vi "Access2DArray.vi"(4 "Sequence Context":T1) -> (0 "error out":errorcluster, 1 "Test Data":T2 {"Numeric Measurement" format="%.2f"})   [LabVIEW 2012]
doc: "This example demonstrates how to use ActiveX to access arrays of data in TestStand from LabVIEW code modules."
uses:
  <vilib>/addons/TestStand/_TSLegacy.llb/LabVIEW Test - Test Data.ctl
  <vilib>/addons/TestStand/_TSLegacy.llb/LabVIEW Test - Sequence Context.ctl
panel:
  out "Array of Data":dbl[][](graph)=[[0.0, 0.12533323356430426, 0.2486898871648548, 0.3681245526846779, 0.4817536741017153, 0.5877852522924731, 0.6845471059286886, 0.7705132427757893, 0.8443279255020151, 0.9048270524660196, 0.9510565162951535, 0.9822872507286886, 0.9980267284282716, 0.9980267284282716, 0.9822872507286887, 0.9510565162951536, 0.9048270524660195, 0.8443279255020152, 0.7705132427757893, 0.6845471059286888, 0.5877852522924732, 0.4817536741017152, 0.36812455268467814, 0.24868988716485482, 0.12533323356430454, 1.2246063538223773e-16, -0.12533323356430429, -0.24868988716485457, -0.3681245526846779, -0.481753674101715, -0.587785252292473, -0.6845471059286887, -0.7705132427757894, -0.8443279255020149, -0.9048270524660194, -0.9510565162951535, -0.9822872507286887, -0.9980267284282716, -0.9980267284282716, -0.9822872507286887, -0.9510565162951536, -0.9048270524660196, -0.844327925502015, -0.7705132427757896, -0.684547105928689, -0.5877852522924734, -0.4817536741017153, -0.36812455268467786, -0.24868988716485535, -0.12533323356430465, -2.4492127076447545e-16, 0.12533323356430418, 0.24868988716485488, 0.36812455268467736, 0.4817536741017149, 0.5877852522924729, 0.6845471059286886, 0.7705132427757893, 0.8443279255020147, 0.9048270524660194, 0.9510565162951535, 0.9822872507286886, 0.9980267284282716, 0.9980267284282716, 0.9822872507286886, 0.9510565162951536, 0.90482705246602, 0.8443279255020151, 0.7705132427757897, 0.6845471059286884, 0.5877852522924734, 0.4817536741017162, 0.368124552684678, 0.2486898871648555, 0.1253332335643039, 3.673819061467132e-16, -0.12533323356430318, -0.24868988716485477, -0.36812455268467725, -0.48175367410171555, -0.5877852522924728, -0.6845471059286878, -0.7705132427757893, -0.8443279255020146, -0.9048270524660197, -0.9510565162951534, -0.9822872507286885, -0.9980267284282716, -0.9980267284282716, -0.9822872507286886, -0.9510565162951538, -0.90482705246602, -0.8443279255020151, -0.7705132427757897, -0.6845471059286885, -0.5877852522924735, -0.4817536741017163, -0.3681245526846781, -0.2486898871648556, -0.125333233564304], [1.0, 0.9921147013144779, 0.9685831611286311, 0.9297764858882515, 0.8763066800438636, 0.8090169943749475, 0.7289686274214116, 0.6374239897486897, 0.5358267949789965, 0.42577929156507266, 0.30901699437494745, 0.18738131458572474, 0.06279051952931353, -0.0627905195293134, -0.1873813145857246, -0.30901699437494734, -0.4257792915650727, -0.5358267949789964, -0.6374239897486897, -0.7289686274214113, -0.8090169943749473, -0.8763066800438636, -0.9297764858882513, -0.9685831611286311, -0.9921147013144778, -1.0, -0.9921147013144779, -0.9685831611286312, -0.9297764858882515, -0.8763066800438637, -0.8090169943749476, -0.7289686274214116, -0.6374239897486895, -0.5358267949789971, -0.42577929156507294, -0.30901699437494756, -0.18738131458572463, -0.06279051952931321, 0.06279051952931283, 0.18738131458572427, 0.30901699437494723, 0.4257792915650726, 0.5358267949789968, 0.6374239897486893, 0.7289686274214112, 0.8090169943749473, 0.8763066800438636, 0.9297764858882515, 0.968583161128631, 0.9921147013144778, 1.0, 0.9921147013144779, 0.9685831611286311, 0.9297764858882517, 0.8763066800438638, 0.8090169943749476, 0.7289686274214116, 0.6374239897486896, 0.5358267949789972, 0.42577929156507305, 0.30901699437494773, 0.18738131458572474, 0.06279051952931332, -0.06279051952931271, -0.18738131458572502, -0.3090169943749471, -0.4257792915650717, -0.5358267949789967, -0.6374239897486892, -0.7289686274214118, -0.8090169943749472, -0.876306680043863, -0.9297764858882515, -0.968583161128631, -0.9921147013144779, -1.0, -0.992114701314478, -0.9685831611286311, -0.9297764858882517, -0.8763066800438635, -0.8090169943749477, -0.7289686274214123, -0.6374239897486897, -0.5358267949789972, -0.4257792915650724, -0.30901699437494784, -0.18738131458572574, -0.06279051952931344, 0.0627905195293126, 0.1873813145857249, 0.309016994374947, 0.4257792915650716, 0.5358267949789965, 0.6374239897486891, 0.7289686274214117, 0.8090169943749471, 0.876306680043863, 0.9297764858882513, 0.968583161128631, 0.9921147013144779]]
  in  "stop":bool
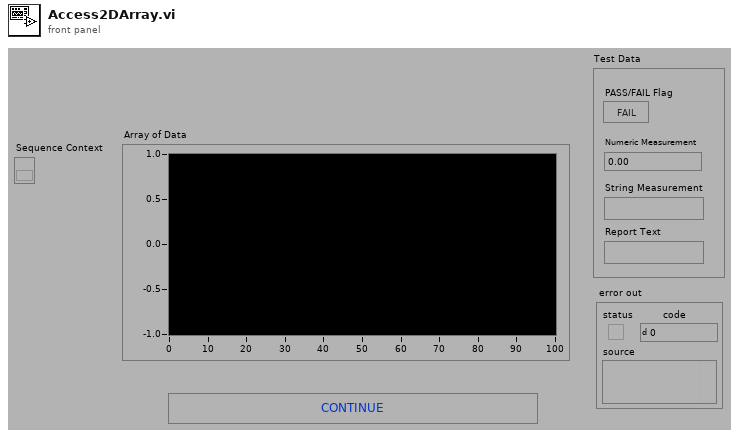
[diagram p1: front panel]
types:
  T1 = typedef "LabVIEW Test - Sequence Context.ctl" = refnum<k7>
  T2 = typedef "LabVIEW Test - Test Data.ctl" = cluster{"PASS/FAIL Flag":bool, "Numeric Measurement":dbl, "String Measurement":string, "Report Text":string}
  T3 = cluster{"Execution":refnum<k7>, "InitTerminationMonitor":refnum<k7>, "Sequence Context Out":refnum<k7>}
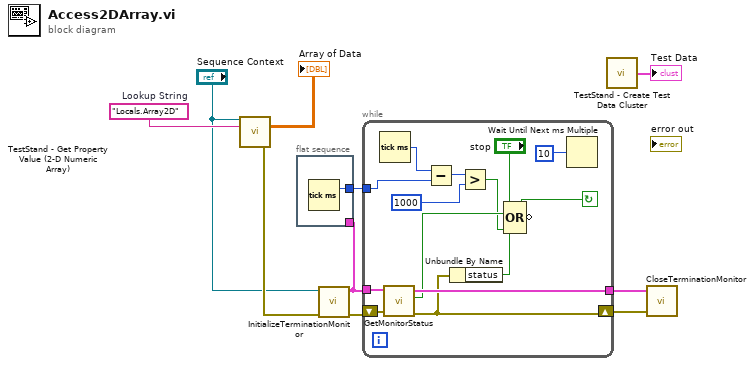
[diagram p0: block diagram]
diagram:
  w9 = "Locals.Array2D"  # Lookup String
  n1 = call "TestStand - Get Property Value (2-D Numeric Array).vi"("Sequence Context In"="Sequence Context", "Lookup String"=w9) -> ("Value"=→"Array of Data":dbl[][], "error out"=w4:errorcluster)  [unwired: 2 in, 10 out]
  n2 = flat-sequence {
    tunnel: [w11] -> w2
    tunnel: w1 -> [_]
    frame #0 {
      n3 = Tick Count (ms)() -> (millisecond timer value=w11:u32)
    }
  }
  n4 = call <vilib>:"InitializeTerminationMonitor.vi"("error in (no error)"=w4, "Sequence Context In"="Sequence Context") -> ("error out"=w7:errorcluster, "StatusMonitor Out"=w1:T3)  [unwired: 8 out]
  n5 = while {
    tunnel: w1 -> [w23]
    tunnel: [w24] -> w5
    shift-left: w7 -> [w25]
    shift-right: [w22] -> w6
    tunnel: w2 -> [w14]
    stop <- w18 continue-if-true
    n6 = Tick Count (ms)() -> (millisecond timer value=w16:u32)
    n7 = call <vilib>:"GetMonitorStatus.vi"("error in"=w25, "StatusMonitor In"=w23) -> ("error out"=w22:errorcluster, "GetTerminationMonitorStatus"=w20:bool, "StatusMonitor Out"=w24:T3)  [unwired: 3 out]
    n8 = Subtract(x=w16, y=w14) -> (x-y=w15:u32)
    n9 = Unbundle By Name(w22) -> ("status"=w19:bool)
    n10 = Greater?(x=w15, y=u32 1000) -> (0:w13:bool)
    n11 = Compound Arithmetic op=OR("stop", w20, w19, w13) -> (invert w18:bool)
    n12 = Wait Until Next ms Multiple(millisecond multiple=u32 10) -> ()  [unwired: 1 out]
  }
  n13 = call <vilib>:"TestStand - Create Test Data Cluster.vi"() -> ("Test Data"=→"Test Data":T2)  [unwired: 4 in]
  n14 = call <vilib>:"CloseTerminationMonitor.vi"("error in"=w6, "StatusMonitor In"=w5) -> ()  [unwired: 4 out]
